vi "Read Configuration.vi"(7 "Section (default)":string, 8 "error in (no error)":errorcluster, 11 "Platano in":refnum<class "Platano.lvclass">) -> (0 "error out":errorcluster, 2 "Config Map":map{string, string}(c390), 3 "Platano out":refnum<class "Platano.lvclass">)   [LabVIEW 2021, in "Bananas.lvlib" / "Platano.lvclass"]
uses:
  Platano.lvclass
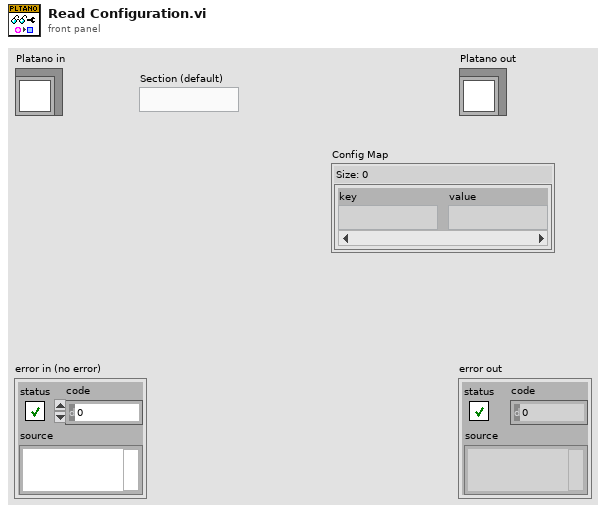
[diagram p1: front panel]
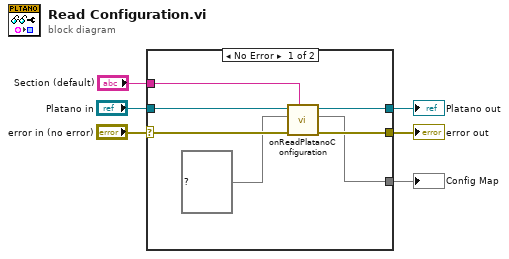
[diagram p0: block diagram]
diagram:
  n1 = case shown="No Error" "error in (no error)" {
    selector: "error in (no error)" -> [w13 w15]
    tunnel: [w12 w15] -> w5
    tunnel: [w8 w14] -> w3
    tunnel: "Platano in" -> [w9 w14]
    tunnel: [w10 _] -> w2
    tunnel: "Section (default)" -> [w7 _]
    frame No Error {
      n2 = call-dynamic "onReadPlatanoConfiguration.vi"("Section (default)"=w7, "error in (no error)"=w13, "Config Map in"=map{string, string} {} ("Config Map"), "Platano in"=w9) -> ("error out"=w12:errorcluster, "Config Map out"=w10:map{string, string}, "Platano out"=w8:refnum<class "Platano.lvclass">)  [unwired: 5 in]
    }
    frame Error {
    }
  }
  "error out" <- w5
  "Platano out" <- w3
  "Config Map" <- w2
